vi "Close Digital and Analog devices.vi"(8 "error in":errorcluster, 9 "analog task":refnum<k21>, 10 "master clock task":T1, 11 "digital audio task":T1) -> (0 "error out":errorcluster)   [LabVIEW 2021]
uses:
  <vilib>/PDM Acquisition Toolkit/host/Classes/Tasks/PCM Output/Controls/PCM Output Task DVR.ctl
  <vilib>/PDM Acquisition Toolkit/host/Classes/Tasks/PCM Output/PCM Output Task.lvclass
  <vilib>/PDM Acquisition Toolkit/host/API/PDM Acquisition Toolkit.lvlib
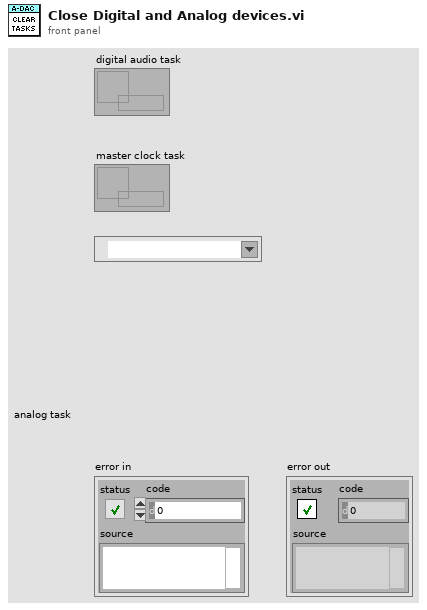
[diagram p1: front panel]
types:
  T1 = typedef "PDM Acquisition Class Library.lvlib/PCM Output Task.lvclass/PCM Output Task DVR.ctl" = refnum<data-value>
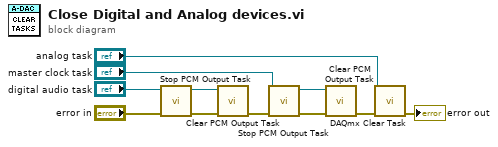
[diagram p0: block diagram]
diagram:
  n1 = call <vilib>:"Stop PCM Output Task.vi"("error in"="error in", "PCM output task In"="digital audio task") -> ("error out"=w8:errorcluster, "PCM output task out"=w9:T1)  [unwired: 8 in]
  n2 = call <vilib>:"Clear PCM Output Task.vi"("error in"=w8, "PCM output task in"=w9) -> ("error out"=w5:errorcluster)  [unwired: 9 in]
  n3 = call <vilib>:"Stop PCM Output Task.vi"("error in"=w5, "PCM output task In"="master clock task") -> ("error out"=w11:errorcluster, "PCM output task out"=w10:T1)  [unwired: 8 in]
  n4 = call <vilib>:"Clear PCM Output Task.vi"("error in"=w11, "PCM output task in"=w10) -> ("error out"=w4:errorcluster)  [unwired: 9 in]
  n5 = call <vilib>:"DAQmx Clear Task.vi"("task in"="analog task", "error in"=w4) -> ("error out"=→"error out":errorcluster)  [unwired: 13 in]
